vi "rad_Open System Config Session.bak.vi"(6 "Timeout ms (4000)":u32=4000, 7 "Access requirement (admin unless unlocked)":T3=enum."Admin unless unlocked", 8 "error in (no error)":errorcluster, 11 "Target settings":T1={"Hostname"="", "Serial number"="", "Product name"="", "Product code"=0, "System status"="", "Credential type"=enum."None/Unlocked", "User added?"=FALSE, "Primary NIC"={"MAC address"="", "IP Address Request Mode"=2, "IP address"="", "Subnet mask"="", "Gateway"="", "DNS server"=""}} {"Primary NIC"."IP Address Request Mode" items=["Static"=1, "DHCP/Link-Local"=2, "Link-Local Only"=4, "DHCP Only"=8]}) -> (0 "error out":errorcluster, 1 "Password out":string, 2 "Cancelled":bool, 3 "Session out":refnum<k21>)   [LabVIEW 2013]
uses:
  Targets/TypeDefs/rad_Initialize Access Types.ctl
  Targets/TypeDefs/rad_Target Information.ctl
  Targets/TypeDefs/rad_Target Network Settings.ctl
  <vilib>/nisyscfg/Close (System).vi
  <vilib>/nisyscfg/nisyscfg.lvlib
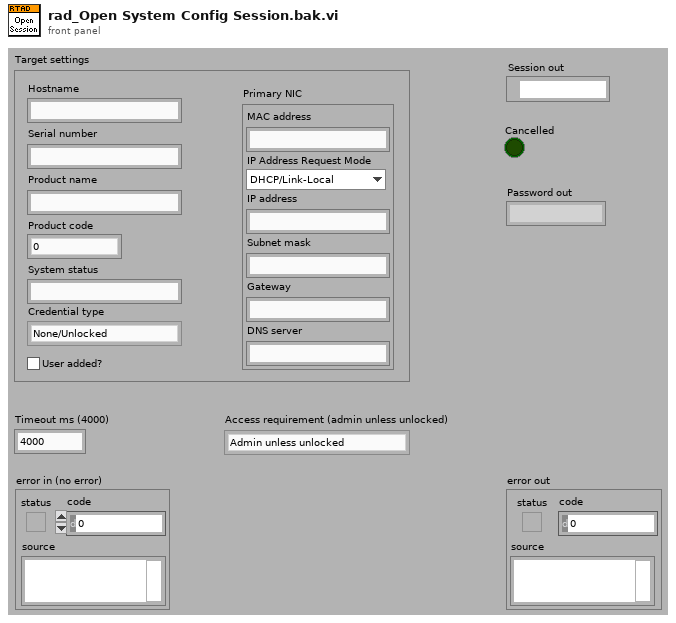
[diagram p1: front panel]
types:
  T1 = typedef "rad_Target Information.ctl" = cluster{"Hostname":string, "Serial number":string, "Product name":string, "Product code":i32, "System status":string, "Credential type":enum16{"None/Unlocked", "FTP Password", "NIAuth Credentials"}, "User added?":bool, "Primary NIC":T2}
  T2 = typedef "rad_Target Network Settings.ctl" = cluster{"MAC address":string, "IP Address Request Mode":i32, "IP address":string, "Subnet mask":string, "Gateway":string, "DNS server":string}
  T3 = typedef "rad_Initialize Access Types.ctl" = enum16{"Anonymous read-only", "Admin unless unlocked", "Admin always"}
  T4 = enum16{"None/Unlocked", "FTP Password", "NIAuth Credentials"}
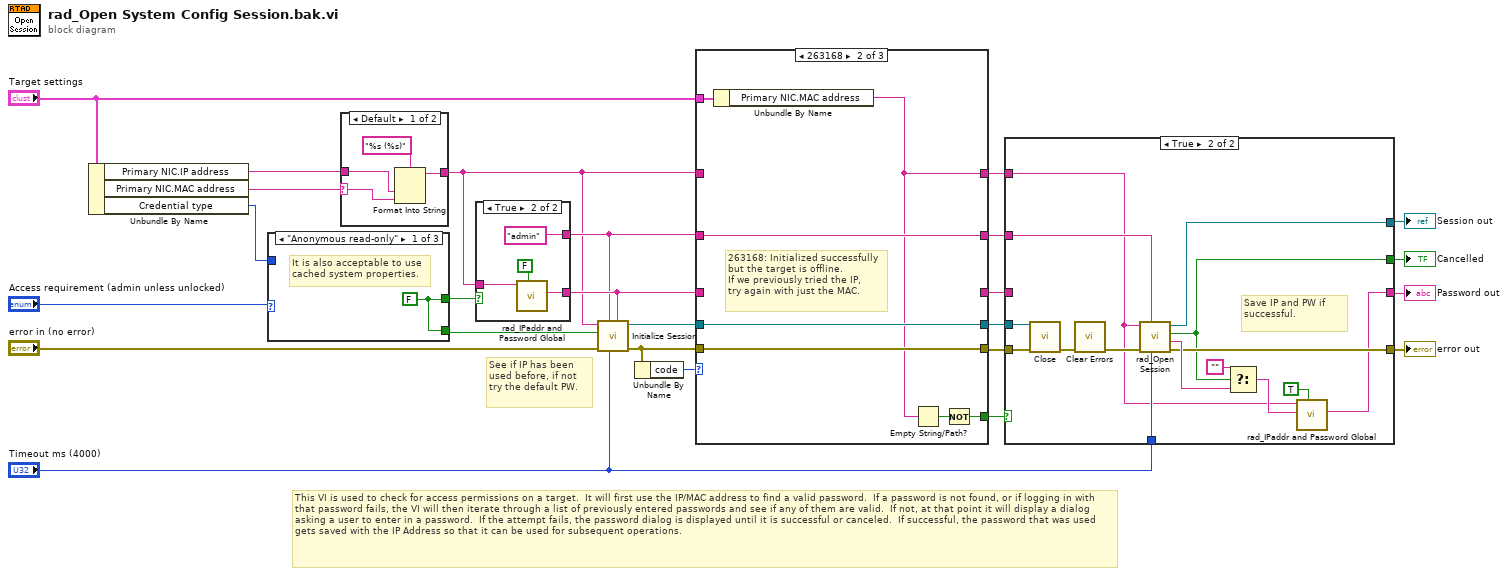
[diagram p0: block diagram]
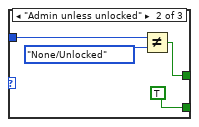
[diagram p3: hidden frame]
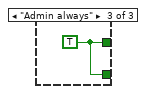
[diagram p4: hidden frame]
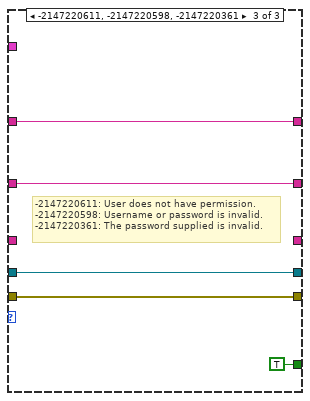
[diagram p8: hidden frame]
diagram:
  # "This VI is used to check for access permissions on a target.  It will first use the IP/MAC address to find a valid password.  If a password is not found, or if logging in with that password fails, the VI will then iterate through a list of previously entered passwords and see if any of them are valid.  If not, at that point it will display a dialog asking a user to enter in a password.  If the attempt fails, the password dialog is displayed until it is successful or canceled.  If successful, the password that was used gets saved with the IP Address so that it can be used for subsequent operations."
  # "See if IP has been used before, if not try the default PW."
  n1 = Unbundle By Name("Target settings") -> ("Primary NIC.IP address"=w13:string, "Primary NIC.MAC address"=w20:string, "Credential type"=w16:T4)
  n2 = case shown="\"Anonymous read-only\"" "Access requirement (admin unless unlocked)" {
    tunnel: w16 -> [_ w29 _]
    tunnel: [w26 w28 w31] -> w15
    tunnel: [w26 TRUE w31] -> w14
    frame "Anonymous read-only" {
      w26 = FALSE
      # "It is also acceptable to use\ncached system properties."
    }
    frame "Admin unless unlocked" {
      n3 = Not Equal?(x=w29, y=T4."None/Unlocked") -> (x != y?=w28:bool)
    }
    frame "Admin always" {
      w31 = TRUE
    }
  }
  n4 = case shown="Default" w20 {
    selector: w20 -> [w33 _]
    tunnel: w13 -> [w34 w36]
    tunnel: [w32 w36] -> w18
    frame Default {
      n5 = Format Into String(format string="%s (%s)", w34, w33) -> (resulting string=w32:string)  [unwired: 2 in, 1 out]
    }
    frame "" {
    }
  }
  n6 = case shown="True" w15 {
    tunnel: [_ w39] -> w21
    tunnel: w18 -> [_ w38]
    tunnel: [_ "admin"] -> w19
    frame False {
    }
    frame True {
      n7 = call "rad_IPaddr and Password Global.vi"("Read(F)/Write(T)"=FALSE, "IP/MAC Address"=w38) -> ("Password"=w39:string)  [unwired: 8 in, 1 out]
    }
  }
  n8 = call <vilib>:"Initialize Session.vi"("Password"=w21, "Connect Timeout (4000 ms)"="Timeout ms (4000)", "User Name"=w19, "error in (no error)"="error in (no error)", "Force Property Refresh (T)"=w14, "Target (localhost)"=w18) -> ("error out"=w24:errorcluster, "Session out"=w23:refnum<k21>)  [unwired: 4 in]
  n9 = Unbundle By Name(w24) -> ("code"=w25:i32)
  n10 = case shown="263168" w25 {
    tunnel: w24 -> [w43 w48 w54]
    tunnel: [w43 w48 w54] -> w11
    tunnel: w23 -> [w41 w49 w53]
    tunnel: w18 -> [_ _ w55]
    tunnel: [w42 _ _] -> w5
    tunnel: w21 -> [w42 _ _]
    tunnel: w19 -> [_ w50 w52]
    tunnel: "Target settings" -> [_ w47 _]
    tunnel: [_ w45 TRUE] -> w12
    tunnel: [_ w44 w55] -> w2
    tunnel: [w41 w49 w53] -> w4
    tunnel: [_ w50 w52] -> w3
    frame Default {
    }
    frame 263168 {
      # "263168: Initialized successfully\nbut the target is offline.\nIf we previously tried the IP,\ntry again with just the MAC."
      n11 = Unbundle By Name(w47) -> ("Primary NIC.MAC address"=w44:string)
      n12 = Empty String/Path?(string/path=w44) -> (empty?=w46:bool)
      n13 = Not(x=w46) -> (.not. x?=w45:bool)
    }
    frame -2147220611, -2147220598, -2147220361 {
      # "-2147220611: User does not have permission.\n-2147220598: Username or password is invalid.\n-2147220361: The password supplied is invalid."
    }
  }
  n14 = case shown="True" w12 {
    tunnel: [w58 w66] -> w7
    tunnel: [w56 w67] -> w10
    tunnel: [w57 w65] -> w8
    tunnel: [_ w64] -> w9
    tunnel: w11 -> [w58 w63]
    tunnel: "Timeout ms (4000)" -> [_ w62]
    tunnel: w5 -> [w57 _]
    tunnel: w4 -> [w56 w61]
    tunnel: w3 -> [_ w60]
    tunnel: w2 -> [_ w59]
    frame False {
    }
    frame True {
      # "Save IP and PW if successful."
      n15 = call-poly <vilib>:"Close.vi"("error in (no error)"=w63, "Session in"=w61) -> ("error out"=w73:errorcluster)  [unwired: 9 in]
      n16 = call <vilib>:"Clear Errors.vi"("error in (no error)"=w73) -> ("error out"=w72:errorcluster)  [unwired: 6 in]
      n17 = call "rad_Open Session.vi"("Timeout ms (4s)"=w62, "User name"=w60, "error in (no error)"=w72, "Target Address"=w59) -> ("error out"=w66:errorcluster, "Password Out"=w70:string, "Cancelled"=w64:bool, "session out"=w67:refnum<k21>)  [unwired: 4 in]
      n18 = Select(t="", s=w64, f=w70) -> (s? t:f=w69:string)
      n19 = call "rad_IPaddr and Password Global.vi"("Read(F)/Write(T)"=TRUE, "Password"=w69, "IP/MAC Address"=w59) -> ("Password"=w65:string)  [unwired: 7 in, 1 out]
    }
  }
  "error out" <- w7
  "Session out" <- w10
  "Cancelled" <- w9
  "Password out" <- w8
